vi "0055 Case arrel quadrada strings.vi"() -> ()   [LabVIEW 2019]
panel:
  out "String":string="error"
  in  "stop":bool
  in  "Entra nombre":dbl
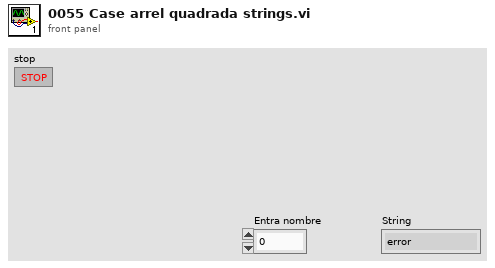
[diagram p1: front panel]
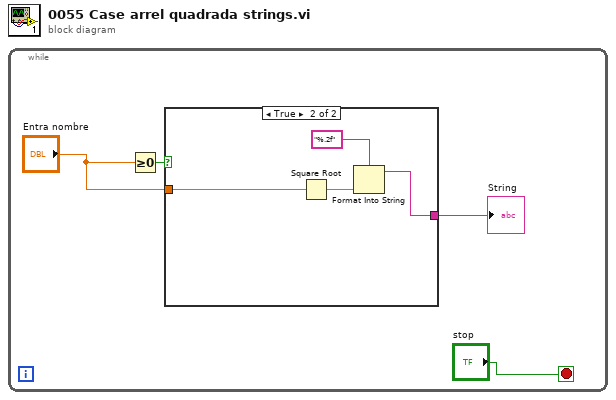
[diagram p0: block diagram]
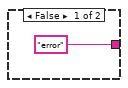
[diagram p2: hidden frame]
diagram:
  n1 = while {
    stop <- "stop" stop-if-true
    n2 = Greater Or Equal To 0?(x="Entra nombre") -> (x >= 0?=w4:bool)
    n3 = case shown="True" w4 {
      tunnel: "Entra nombre" -> [_ w9]
      tunnel: ["error" w7] -> w1
      frame False {
      }
      frame True {
        n4 = Square Root(x=w9) -> (sqrt(x)=w8:dbl)
        n5 = Format Into String(format string="%.2f", w8) -> (resulting string=w7:string)  [unwired: 2 in, 1 out]
      }
    }
    "String" <- w1
  }
